vi "Read CSV file.vi"(1 "decimal mark":string=".", 2 "file path (dialog if empty)":path=path "C:/Users/primo_000/Documents/LabVIEW Data/test.txt", 4 "delimiter (,)":string=",") -> (16 "row":dbl[](array[numeric]) format="%0.3f")   [LabVIEW 2010, in "RedPitaya.lvlib"]
doc: "Reads CSV file definded by <b>file path</b>. You can also set <b>delimiter</b> and <b>decimal mark</b> for reading text file. You can use values from <b> -1 to +1</b>\n\nOn defailt settings the CSV file should be built like this:\n0.54,-0.164,0.667,-0.156,0.754,-0.13"
uses:
  RedPitaya.lvlib
  <vilib>/Utility/file.llb/Read From Spreadsheet File (DBL).vi
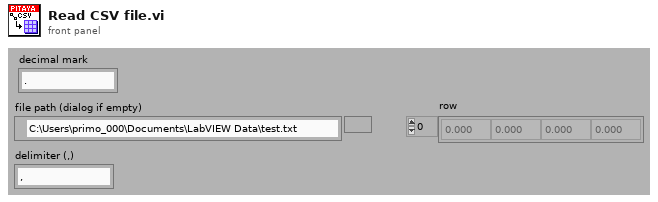
[diagram p1: front panel]
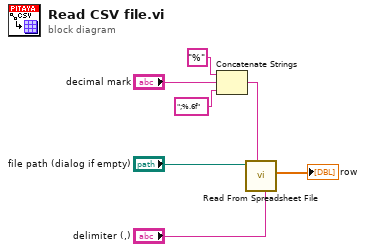
[diagram p0: block diagram]
diagram:
  n1 = Concatenate Strings("%" ("format (%.3f)"), "decimal mark", ";%.6f" ("format (%.3f)")) -> (w2:string)
  n2 = call-poly <vilib>:"Read From Spreadsheet File.vi"("delimiter (\\t)"="delimiter (,)", "format (%.3f)"=w2, "file path (dialog if empty)"="file path (dialog if empty)") -> ("first row"=→"row":dbl[])  [unwired: 4 in, 4 out]
